vi "PythonNode_ComputeCrossProduct.vi"() -> ()   [LabVIEW 2023]
uses:
  support/PythonVersionsEnum_Namedtuples.ctl
panel:
  out "vector1 X vector2":cluster{"i":i32, "j":i32, "k":i32}
  in  "vector 2":cluster{"i":i32, "j":i32, "k":i32}={"i"=2, "j"=-3, "k"=1}
  in  "python version":T1
  in  "vector 1":cluster{"i":i32, "j":i32, "k":i32}={"i"=1, "j"=2, "k"=-1}
  out "error out":errorcluster
  in  "error in (no error)":errorcluster
  # "Overview: Demonstrates how to call a Python function, pass labeled clusters as python namedtuples (arguments) and accept python namedtuples as labeled clusters(return value).\nRequirements: Python 3.8, 3.9 or 3.10 with the same bitness as LabVIEW.\nInstructions:\n1. Set the Python version to the version of Python you want to execute code in.\n2. Run the VI. You should see the result as the cross product of \"vector 1\" and \"vector 2\" in the indicator \"vector 1 X vector 2\".\n3. See comments on the block diagram of this VI and in \"ExamplePythonModule.py\" for more information about how the call python node passes arguments and handles return values."
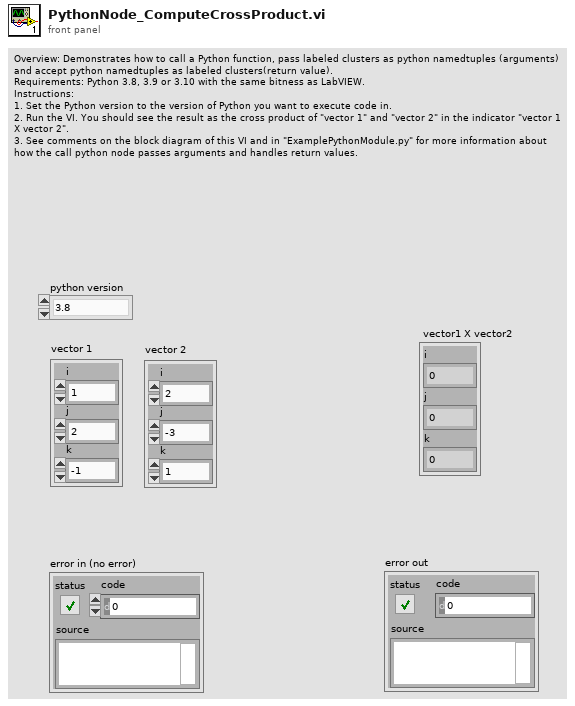
[diagram p1: front panel]
types:
  T1 = typedef "PythonVersionsEnum_Namedtuples.ctl" = enum16{"3.8", "3.9", "3.10"}
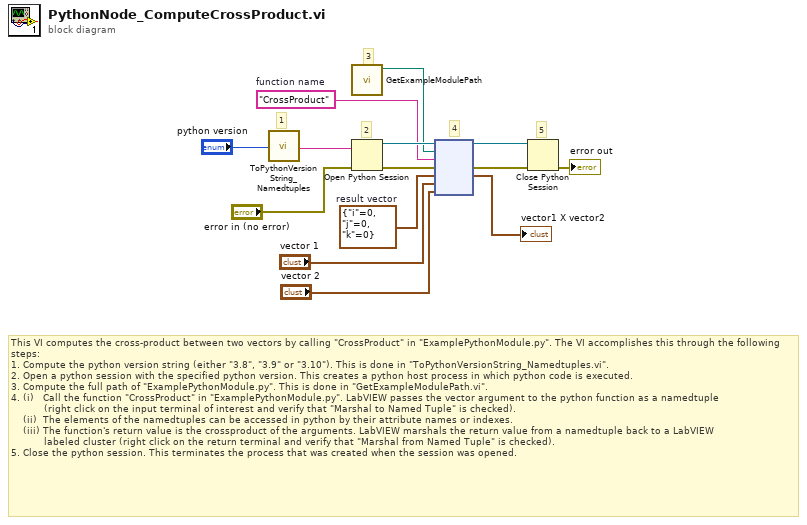
[diagram p0: block diagram]
diagram:
  w5 = cluster{"i":i32, "j":i32, "k":i32} {"i"=0, "j"=0, "k"=0}  # result vector
  w10 = "CrossProduct"  # function name
  # "This VI computes the cross-product between two vectors by calling \"CrossProduct\" in \"ExamplePythonModule.py\". The VI accomplishes this through the following steps:\n1. Compute the python version string (either \"3.8\", \"3.9\" or \"3.10\"). This is done in \"ToPythonVersionString_Namedtuples.vi\". \n2. Open a python session with the specified python version. This creates a python host process in which python code is executed.\n3. Compute the full path of \"ExamplePythonModule.py\". This is done in \"GetExampleModulePath.vi\".\n4. (i)   Call the function \"CrossProduct\" in \"ExamplePythonModule.py\". LabVIEW passes the vector argument to the python function as a namedtuple\n           (right click on the input terminal of interest and verify that \"Marshal to Named Tuple\" is checked). \n    (ii)  The elements of the namedtuples can be accessed in python by their attribute names or indexes.       \n    (iii) The function's return value is the crossproduct of the arguments. LabVIEW marshals the return value from a namedtuple back to a LabVIEW  \n           labeled cluster (right click on the return terminal and verify that \"Marshal from Named Tuple\" is checked). \n5. Close the python session. This terminates the process that was created when the session was opened."
  # "5"
  # "4"
  # "2"
  # "3"
  # "1"
  n1 = call "ToPythonVersionString_Namedtuples.vi"("python version"="python version") -> ("python version string"=w4:string)  [unwired: 10 in]
  n2 = call "GetExampleModulePath.vi"() -> ("module path"=w11:path)  [unwired: 11 in]
  n3 = Open Python Session(python version=w4, 3:"error in (no error)") -> (session out=w13:refnum<k35>, error out=w12:errorcluster)  [unwired: 1 in]
  n4 = node(w13, w11, w10, w12, w5, "vector 1", "vector 2") -> (w9:refnum<k35>, w8:errorcluster, →"vector1 X vector2":cluster{"i":i32, "j":i32, "k":i32})  [unwired: 2 in, 2 out]
  n5 = Close Python Session(session in=w9, error in=w8) -> (11:→"error out":errorcluster)
